vi "FestoCPX.booleanToFrameValve.vi"(10 "Raw Array":bool[](array[boolean])) -> (2 "Bytes DO":u8[](array[numeric]))   [LabVIEW 2013]
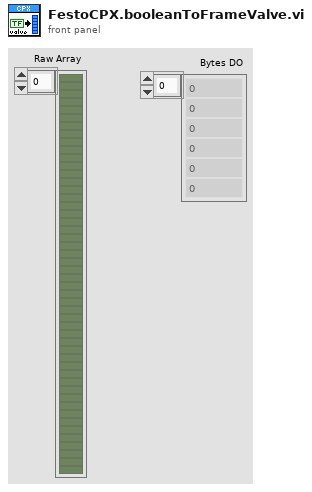
[diagram p1: front panel]
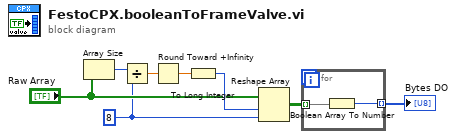
[diagram p0: block diagram]
diagram:
  w1 = 8 ("dimension size")
  n1 = Array Size(array="Raw Array") -> (size(s)=w8:i32)
  n2 = Divide(x=w8, y=w1) -> (x/y=w7:dbl)
  n3 = Round Toward +Infinity(x=w7) -> (ceil(x): smallest int >= x=w6:dbl)
  n4 = To Long Integer(number=w6) -> (32bit integer=w4:i32)
  n5 = Reshape Array("Raw Array", w4, w1) -> (w5:bool[][])
  n6 = for {
    tunnel: w5 -> [w10] mode=indexing
    tunnel: [w9] -> w3 mode=indexing
    n7 = Boolean Array To Number(Boolean array=w10) -> (number=w9:u8)
  }
  "Bytes DO" <- w3
